vi "Initialize Redis TCP Client.vi"(7 "Redis TCP Client in":refnum<class "Redis TCP Client.lvclass">, 8 "error in (no error)":errorcluster, 9 "timeout ms (25000)":i32=25000, 10 "remote port or service name":u16=6379, 11 "address":string) -> (0 "error out":errorcluster, 3 "Redis TCP Client out":refnum<class "Redis TCP Client.lvclass">)   [LabVIEW 2019, in "Redis Client for LabVIEW.lvlib" / "Redis TCP Client.lvclass"]
uses:
  Redis TCP Client.lvclass
  lib/RESP3-for-LabVIEW/RESP3/RESP3 Parser/RESP3 Parser.lvclass
  Redis TCP Client.lvclass/Redis TCP Client.ctl
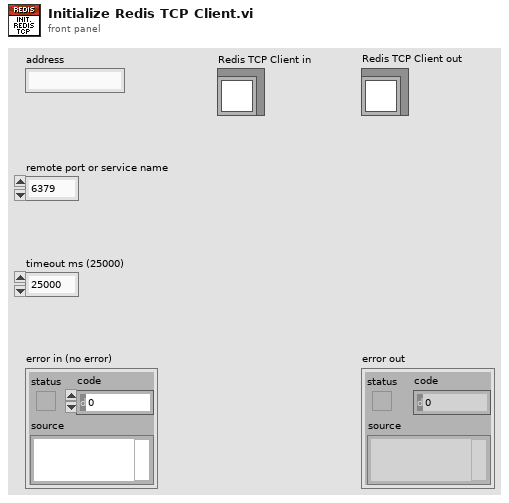
[diagram p1: front panel]
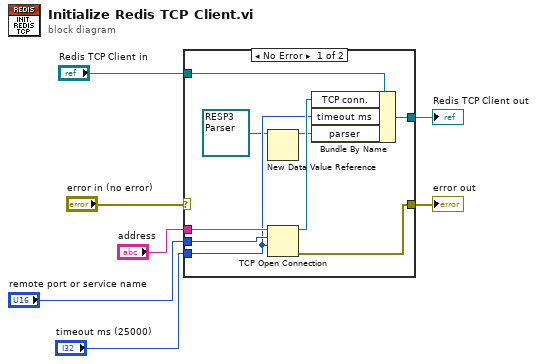
[diagram p0: block diagram]
diagram:
  n1 = case shown="No Error" "error in (no error)" {
    selector: "error in (no error)" -> [_ w18]
    tunnel: [w14 w18] -> w6
    tunnel: [w13 w17] -> w4
    tunnel: "Redis TCP Client in" -> [w12 w17]
    tunnel: "address" -> [w16 _]
    tunnel: "remote port or service name" -> [w15 _]
    tunnel: "timeout ms (25000)" -> [w10 _]
    frame No Error {
      n2 = New Data Value Reference(data value=refnum<class "RESP3 Parser.lvclass"> refnum ("RESP3.lvlib:RESP3 Parser.lvclass")) -> (data value reference=w8:refnum<data-value>)  [unwired: 1 in, 1 out]
      n3 = TCP Open Connection(address=w16, remote port or service name=w15, timeout ms (60000)=w10) -> (connection ID=w11:refnum<k5>, error out=w14:errorcluster)  [unwired: 2 in]
      n4 = Bundle By Name(cluster=w12, "TCP conn."=w11, "timeout ms"=w10, "parser"=w8) -> (w13:refnum<class "Redis TCP Client.lvclass">)
    }
    frame Error {
    }
  }
  "error out" <- w6
  "Redis TCP Client out" <- w4
